vi "scale xy steering.vi"(2 "0 to 9 V input":dbl, 3 "-2.5 to 2.5 V input":dbl) -> (0 "-2.5 to 2.5 V output":dbl, 1 "0 to 9 V output":dbl)   [LabVIEW 2013]
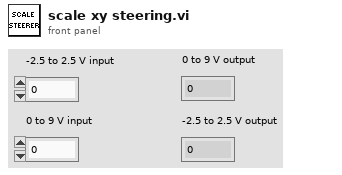
[diagram p1: front panel]
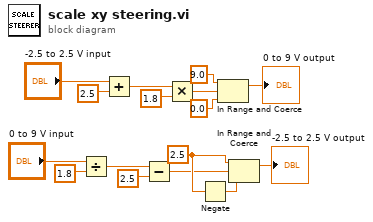
[diagram p0: block diagram]
diagram:
  w8 = 2.5 ("upper limit")
  n1 = Divide(x="0 to 9 V input", y=1.8) -> (x/y=w10:dbl)
  n2 = Add(x="-2.5 to 2.5 V input", y=2.5) -> (x+y=w14:dbl)
  n3 = Subtract(x=w10, y=2.5) -> (x-y=w5:dbl)
  n4 = Multiply(x=w14, y=1.8) -> (x*y=w4:dbl)
  n5 = Negate(x=w8) -> (-x=w7:dbl)
  n6 = In Range and Coerce(upper limit=9.0, x=w4, lower limit=0.0) -> (coerced(x)=→"0 to 9 V output":dbl)  [unwired: 1 out]
  n7 = In Range and Coerce(upper limit=w8, x=w5, lower limit=w7) -> (coerced(x)=→"-2.5 to 2.5 V output":dbl)  [unwired: 1 out]
